vi "Multiplexer.vi"() -> ()   [LabVIEW 2018]
uses:
  <vilib>/Instr/_visa.llb/VISA Configure Serial Port (Instr).vi
panel:
  out "error out":errorcluster
  in  "Tab Control":enum32{"Manual", "Auto"}(tab)
  in  "Send Command":bool
  in  "Multiplexer Command":T1(ring)
  in  "Position":i32
  in  "Time between\nSwitches":u32=2000
  out "Last Sent Position":i32
  in  "stop":bool
  in  "Multiplexer\nPort":refnum<visa-resource-name>="COM16"
  out "Multiplexer Response":string="0"
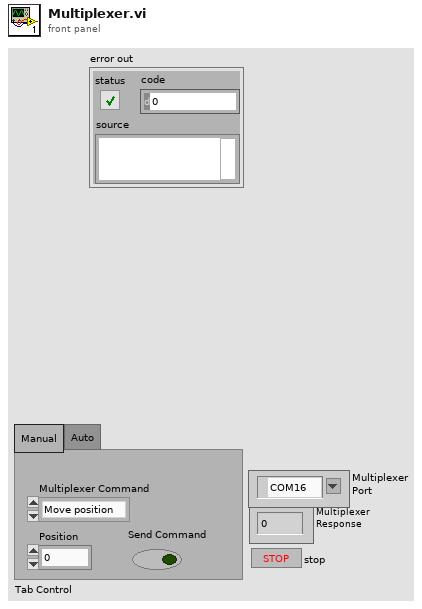
[diagram p1: front panel]
types:
  T1 = enum16{"Move position", "Get Status", "Get Program"}
  T2 = cluster{"baud rate":u32, "data bits":u16, "parity":enum16{"None", "Odd", "Even", "Mark", "Space"}, "stop bits":u16, "flow control":u16}
  T3 = enum32{"Invalid", "Standard", "Closed", "Hidden", "Minimized", "Maximized"}
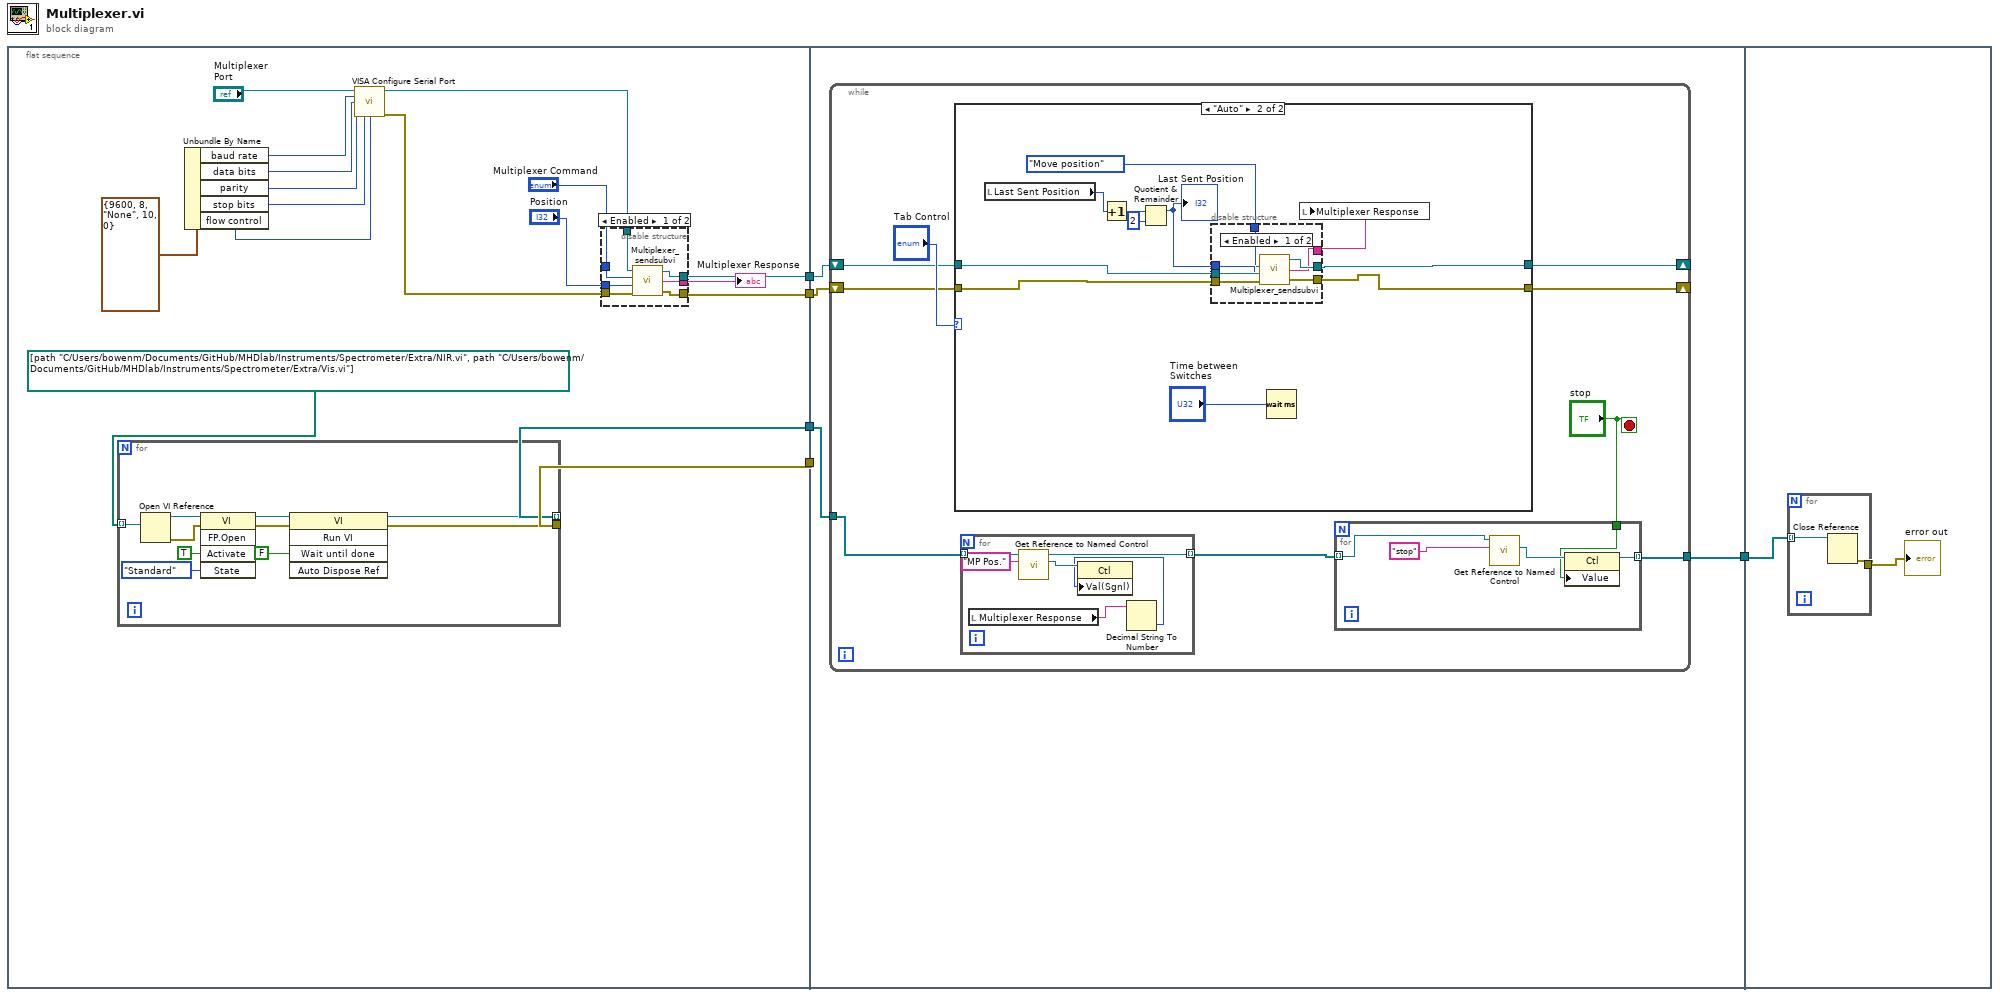
[diagram p0: block diagram]
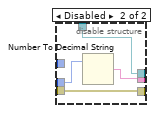
[diagram p2: hidden frame]
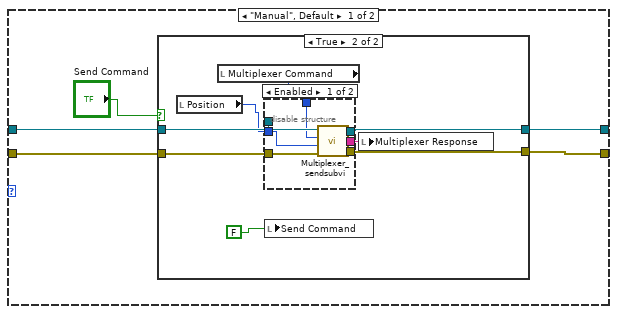
[diagram p3: hidden frame]
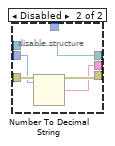
[diagram p5: hidden frame]
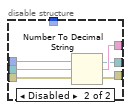
[diagram p6: hidden frame]
diagram:
  n1 = flat-sequence {
    tunnel: [w11] -> w5
    tunnel: [w10] -> w4
    tunnel: [w7] -> w3
    tunnel: [w8] -> w2
    tunnel: w5 -> [w47]
    tunnel: w4 -> [w46]
    tunnel: w3 -> [w45]
    tunnel: w2 -> [_]
    tunnel: [w44] -> w1
    tunnel: w1 -> [w116]
    frame #0 {
      n2 = for {
        tunnel: path[] [path "C:/Users/bowenm/Documents/GitHub/MHDlab/Instruments/Spectrometer/Extra/NIR.vi", path "C:/Users/bowenm/Documents/GitHub/MHDlab/Instruments/Spectrometer/Extra/Vis.vi"] -> [w32] mode=indexing
        tunnel: [w24] -> w7 mode=indexing
        tunnel: [w23] -> w8
        n3 = Open VI Reference(vi path=w32) -> (vi reference=w28:refnum<vi>, error out=w27:errorcluster)  [unwired: 5 in]
        n4 = invoke class="VI" method="FP.Open"(reference=w28, error in=w27, "Activate"=TRUE ("Activate?"), "State"=T3."Standard") -> (reference out=w29:refnum<vi>, error out=w30:errorcluster)  [unwired: 1 in, 3 out]
        n5 = invoke class="VI" method="Run VI"(reference=w29, error in=w30, "Wait until done"=FALSE ("Wait Until Done")) -> (reference out=w24:refnum<vi>, error out=w23:errorcluster)  [unwired: 2 in, 3 out]
      }
      n6 = Unbundle By Name(T2 {"baud rate"=9600, "data bits"=8, "parity"=enum."None", "stop bits"=10, "flow control"=0} ("Serial Settings")) -> ("baud rate"=w20:u32, "data bits"=w19:u16, "parity"=w18:enum16{"None", "Odd", "Even", "Mark", "Space"}, "stop bits"=w17:u16, "flow control"=w16:u16)
      n7 = call-poly "VISA Configure Serial Port"("VISA resource name"="Multiplexer\nPort", "baud rate (9600)"=w20, "data bits (8)"=w19, "parity (0:none)"=w18, "stop bits (10: 1 bit)"=w17, "flow control (0:none)"=w16) -> ("VISA resource name out"=w9:refnum<visa-resource-name>, "error out"=w13:errorcluster)  [unwired: 3 in, 5 out]
      n8 = disable-structure shown="Enabled" {
        disable-tunnel: "Position" -> [w39 w43]
        disable-tunnel: "Multiplexer Command" -> [w38 _]
        disable-tunnel: w13 -> [w37 w41]
        disable-tunnel: w9 -> [w36 w40]
        disable-tunnel: [w35 w42] -> w12
        disable-tunnel: [w34 w40] -> w11
        disable-tunnel: [w33 w41] -> w10
        frame Enabled {
          n9 = call "Multiplexer_sendsubvi.vi"("error in (no error)"=w37, "Position"=w39, "Enum"=w38, "VISA resource name"=w36) -> ("error out"=w33:errorcluster, "Response"=w35:string, "VISA resource name out"=w34:refnum<visa-resource-name>)
        }
        frame Disabled {
          n10 = Number To Decimal String(number=w43) -> (decimal integer string=w42:string)  [unwired: 1 in]
        }
      }
      "Multiplexer Response" <- w12
    }
    frame #1 {
      n11 = while {
        shift-right: [w53] -> _
        shift-left: w47 -> [w55]
        shift-right: [w52] -> _
        shift-left: w46 -> [w54]
        tunnel: w45 -> [w49]
        tunnel: [w50] -> w44
        stop <- "stop" stop-if-true
        n12 = case shown="\"Auto\"" "Tab Control" {
          tunnel: w55 -> [w72 w104]
          tunnel: w54 -> [w71 w103]
          tunnel: [w70 w102] -> w53
          tunnel: [w69 w101] -> w52
          frame "Manual", Default {
            n13 = case shown="True" "Send Command" {
              tunnel: w72 -> [w74 w82]
              tunnel: w71 -> [w73 w81]
              tunnel: [w74 w80] -> w70
              tunnel: [w73 w79] -> w69
              frame False {
              }
              frame True {
                n14 = local read "Position"() -> (w75:i32)
                n15 = local read "Multiplexer Command"() -> (w78:T1)
                n16 = disable-structure shown="Enabled" {
                  disable-tunnel: w82 -> [w89 w92]
                  disable-tunnel: w81 -> [w88 w93]
                  disable-tunnel: [w87 w92] -> w80
                  disable-tunnel: [w86 w93] -> w79
                  disable-tunnel: w75 -> [w85 w90]
                  disable-tunnel: w78 -> [w84 _]
                  disable-tunnel: [w83 w91] -> w77
                  frame Enabled {
                    n17 = call "Multiplexer_sendsubvi.vi"("error in (no error)"=w88, "Position"=w85, "Enum"=w84, "VISA resource name"=w89) -> ("error out"=w86:errorcluster, "Response"=w83:string, "VISA resource name out"=w87:refnum<visa-resource-name>)
                  }
                  frame Disabled {
                    n18 = Number To Decimal String(number=w90) -> (decimal integer string=w91:string)  [unwired: 1 in]
                  }
                }
                n19 = local write "Send Command"(FALSE) -> ()
                n20 = local write "Multiplexer Response"(w77) -> ()
              }
            }
          }
          frame "Auto" {
            n21 = local read "Last Sent Position"() -> (w94:i32)
            n22 = Increment(x=w94) -> (x+1=w97:i32)
            n23 = Quotient & Remainder(x=w97, y=2) -> (x-y*floor(x/y)=w95:i32)  [unwired: 1 out]
            "Last Sent Position" <- w95
            n24 = disable-structure shown="Enabled" {
              disable-tunnel: w95 -> [w106 w115]
              disable-tunnel: T1."Move position" ("Multiplexer Command 2") -> [w105 _]
              disable-tunnel: w104 -> [w111 w112]
              disable-tunnel: w103 -> [w110 w114]
              disable-tunnel: [w109 w112] -> w102
              disable-tunnel: [w108 w114] -> w101
              disable-tunnel: [w107 w113] -> w98
              frame Enabled {
                n25 = call "Multiplexer_sendsubvi.vi"("error in (no error)"=w110, "Position"=w106, "Enum"=w105, "VISA resource name"=w111) -> ("error out"=w108:errorcluster, "Response"=w107:string, "VISA resource name out"=w109:refnum<visa-resource-name>)
              }
              frame Disabled {
                n26 = Number To Decimal String(number=w115) -> (decimal integer string=w113:string)  [unwired: 1 in]
              }
            }
            n27 = Wait (ms)(milliseconds to wait="Time between\nSwitches") -> ()  [unwired: 1 out]
            n28 = local write "Multiplexer Response"(w98) -> ()
          }
        }
        n29 = for {
          tunnel: w49 -> [w62] mode=indexing
          tunnel: [w61] -> w48 mode=indexing
          n30 = local read "Multiplexer Response"() -> (w58:string)
          n31 = call "Get Reference to Named Control.vi"("Control Name"="MP Pos.", "Front Panel Ref"=w62) -> ("Ctl Refnum"=w59:refnum<vi>, "Panel Ref Out"=w61:refnum<vi>)  [unwired: 7 in, 1 out]
          n32 = Decimal String To Number(string=w58) -> (number=w57:i32)  [unwired: 2 in, 1 out]
          n33 = property class="Ctl"(reference=w59, "Val(Sgnl)"=w57) -> ()  [unwired: 1 in, 2 out]
        }
        n34 = for {
          tunnel: "stop" -> [w66]
          tunnel: w48 -> [w64] mode=indexing
          tunnel: [w63] -> w50 mode=indexing
          n35 = call "Get Reference to Named Control.vi"("Control Name"="stop", "Front Panel Ref"=w64) -> ("Ctl Refnum"=w67:refnum<vi>)  [unwired: 7 in, 2 out]
          n36 = property class="Ctl"(reference=w67, "Value"=w66) -> (reference out=w63:refnum<vi>)  [unwired: 1 in, 1 out]
        }
      }
    }
    frame #2 {
      n37 = for {
        tunnel: [w119] -> w117
        tunnel: w116 -> [w118] mode=indexing
        n38 = Close Reference(reference=w118) -> (error out=w119:errorcluster)  [unwired: 1 in]
      }
      "error out" <- w117
    }
  }
